vi "TEC COM Reconnect.vi"(8 "error in (no error)":errorcluster, 9 "TEC ID":i32, 11 "queue in":refnum<queue>) -> (0 "error out":errorcluster)   [LabVIEW 2020]
uses:
  typedefs/TEC Queue Messages.ctl
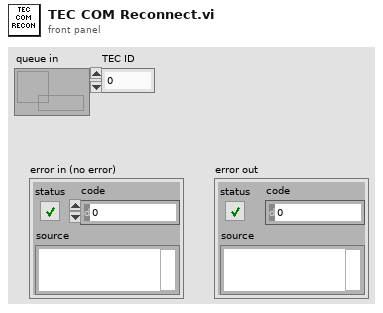
[diagram p1: front panel]
types:
  T1 = typedef "TEC Queue Messages.ctl" = enum16{"Auto Detect", "Connect", "Disconnect", "Exit", "Set Temp", "Output Ena", "RESET"}
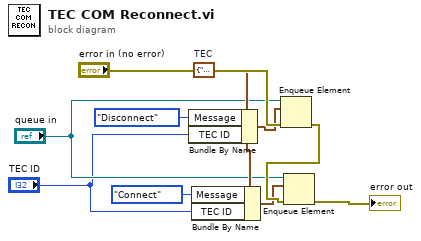
[diagram p0: block diagram]
diagram:
  w7 = cluster{"Message":T1, "TEC ID":i32, "Data":dbl} {"Message"=enum."Connect", "TEC ID"=0, "Data"=0.0}  # TEC
  n1 = Bundle By Name(cluster=w7, "Message"=TEC_Queue_Messages."Disconnect", "TEC ID"="TEC ID") -> (w3:cluster{"Message":T1, "TEC ID":i32, "Data":dbl})
  n2 = Bundle By Name(cluster=w7, "Message"=TEC_Queue_Messages."Connect", "TEC ID"="TEC ID") -> (w2:cluster{"Message":T1, "TEC ID":i32, "Data":dbl})
  n3 = Enqueue Element(queue="queue in", element=w3, error in (no error)="error in (no error)") -> (error out=w8:errorcluster)  [unwired: 1 in, 2 out]
  n4 = Enqueue Element(queue="queue in", element=w2, error in (no error)=w8) -> (error out=→"error out":errorcluster)  [unwired: 1 in, 2 out]
